vi "CalibrateFilters.vi"() -> ()   [LabVIEW 2024]
uses:
  <vilib>/Analysis/baseanly.llb/Mean (DBL).vi
  <instrlib>/Thorlabs_FW102C/Thorlabs_FW102C.lvlib
  <instrlib>/Keithley 648X Series/Keithley 648X Series.lvlib
  <vilib>/Analysis/NI_AALBase.lvlib
panel:
  out "ND":dbl[](array[numeric])
  out "x/y":dbl[](array[numeric])
  out "Position":i32
  out "Avg Pos 0":dbl format="%#_6p"
  out "Connected?":bool
  out "ID":string
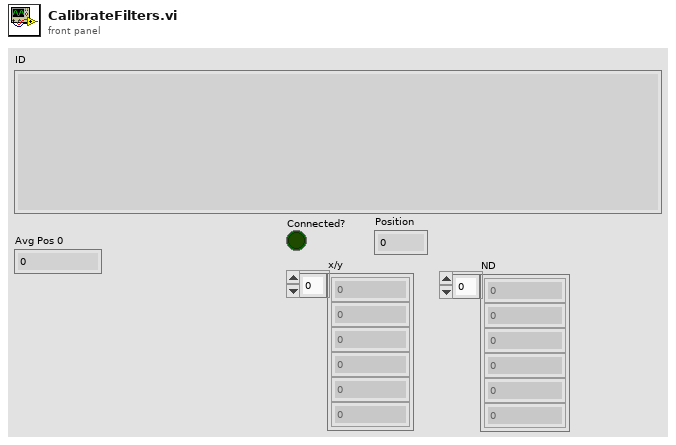
[diagram p1: front panel]
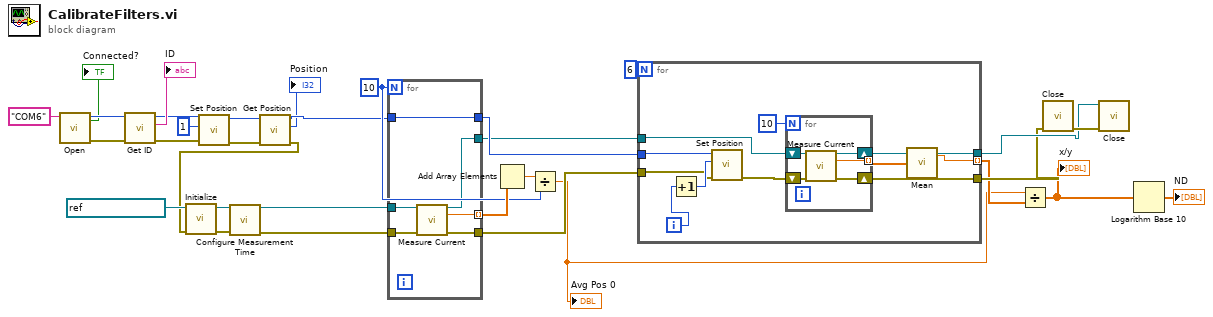
[diagram p0: block diagram]
diagram:
  w17 = 10
  n1 = call <instrlib>:"Open.vi"("Serial Port"="COM6") -> ("error out"=w31:errorcluster, "FW102C out"=w32:i32, "Connected?"=→"Connected?":bool)  [unwired: 8 in]
  n2 = call <instrlib>:"Get ID.vi"("error in (no error)"=w31, "FW102C in"=w32) -> ("error out"=w26:errorcluster, "ID"=→"ID":string, "FW102C out"=w27:i32)  [unwired: 7 in]
  n3 = call <instrlib>:"Set Position.vi"("error in (no error)"=w26, "Position"=1, "FW102C in"=w27) -> ("error out"=w15:errorcluster, "FW102C out"=w14:i32)  [unwired: 7 in]
  n4 = call <instrlib>:"Get Position.vi"("error in (no error)"=w15, "FW102C in"=w14) -> ("error out"=w13:errorcluster, "Position"=→"Position":i32, "FW102C out"=w12:i32)  [unwired: 7 in]
  n5 = call <instrlib>:"Initialize.vi"("error in (no error)"=w13, "VISA resource name"=refnum<visa-resource-name> "Picoammeter") -> ("error out"=w23:errorcluster, "VISA resource name out"=w24:refnum<visa-resource-name>)  [unwired: 8 in]
  n6 = call <instrlib>:"Configure Measurement Time.vi"("VISA resource name"=w24, "error in (no error)"=w23) -> ("VISA resource name out"=w21:refnum<visa-resource-name>, "error out"=w20:errorcluster)  [unwired: 12 in]
  n7 = for {
    N: w17 -> [_]
    tunnel: w21 -> [w38]
    tunnel: w12 -> [w35]
    tunnel: w20 -> [w37]
    tunnel: [w36] -> w19 mode=indexing
    tunnel: [w35] -> w9
    tunnel: [w34] -> w8
    tunnel: [w33] -> w7
    n8 = call <instrlib>:"Measure Current.vi"("VISA resource name"=w38, "error in (no error)"=w37) -> ("VISA resource name out"=w33:refnum<visa-resource-name>, "Measurement"=w36:dbl, "error out"=w34:errorcluster)  [unwired: 11 in]
  }
  n9 = Add Array Elements(numeric array=w19) -> (sum=w18:dbl)
  n10 = Divide(x=w18, y=w17) -> (x/y=w3:dbl)
  "Avg Pos 0" <- w3
  n11 = for {
    N: 6 -> [_]
    tunnel: w9 -> [w49]
    tunnel: w8 -> [w46]
    tunnel: w7 -> [w44]
    tunnel: [w43] -> w6
    tunnel: [w42] -> w5
    tunnel: [w39] -> w4 mode=indexing
    i -> [w48]
    n12 = Increment(x=w48) -> (x+1=w47:i32)
    n13 = call <instrlib>:"Set Position.vi"("error in (no error)"=w46, "Position"=w47, "FW102C in"=w49) -> ("error out"=w45:errorcluster)  [unwired: 7 in, 1 out]
    n14 = for {
      N: 10 -> [_]
      tunnel: [w50] -> w40 mode=indexing
      shift-right: [w51] -> w42
      shift-left: w45 -> [w54]
      shift-right: [w52] -> w43
      shift-left: w44 -> [w53]
      n15 = call <instrlib>:"Measure Current.vi"("VISA resource name"=w53, "error in (no error)"=w54) -> ("VISA resource name out"=w52:refnum<visa-resource-name>, "Measurement"=w50:dbl, "error out"=w51:errorcluster)  [unwired: 11 in]
    }
    n16 = call-poly <vilib>:"Mean.vi"("X"=w40) -> ("mean"=w39:dbl)  [unwired: 1 out]
  }
  n17 = Divide(x=w3, y=w4) -> (x/y=w2:dbl[])
  "x/y" <- w2
  n18 = call <instrlib>:"Close.vi"("error in (no error)"=w5) -> ("error out"=w16:errorcluster)  [unwired: 10 in]
  n19 = call <instrlib>:"Close.vi"("error in (no error)"=w16, "VISA resource name"=w6) -> ()  [unwired: 9 in, 1 out]
  n20 = Logarithm Base 10(1:w2) -> (0:→"ND":dbl[])
